vi "BB_Local Sense Test_v3.vi"(7 "error in (no error)":errorcluster, 10 "Control Board VISA":refnum<visa-resource-name>) -> (0 "error out":errorcluster, 2 "Voltage Readings":dbl[][](array[numeric]), 3 "Pass?":bool)   [LabVIEW 2022 SP3]
panel:
  in  "LocalSenseRelayTask":refnum<k21>="BTS_LocalSenseRelays"
  out "MSE Array":dbl[](array[numeric])
  out "Message OUT":string
  in  "Message IN":string
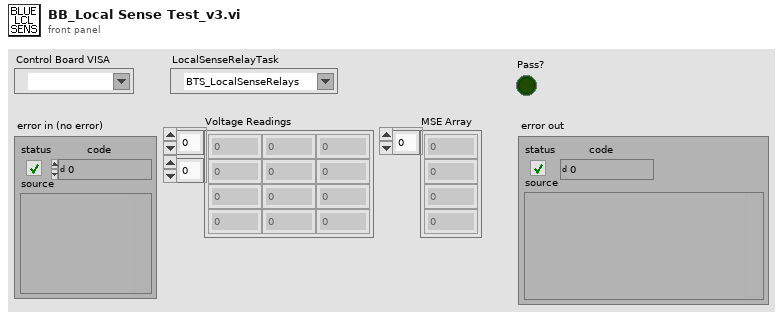
[diagram p1: front panel]
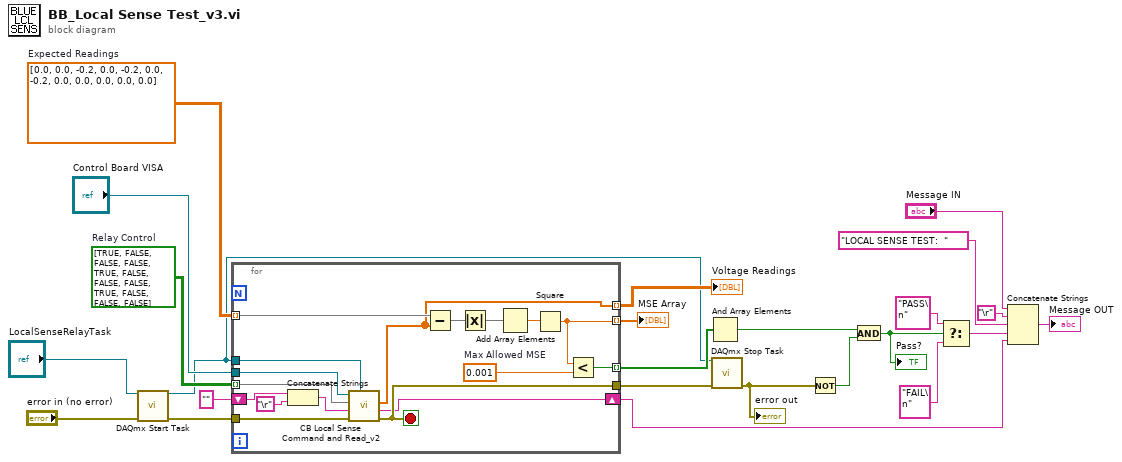
[diagram p0: block diagram]
diagram:
  w7 = dbl[][] [[0.0, 0.0, -0.2], [0.0, -0.2, 0.0], [-0.2, 0.0, 0.0], [0.0, 0.0, 0.0]]  # Expected Readings
  w23 = bool[][] [[TRUE, FALSE, FALSE], [FALSE, TRUE, FALSE], [FALSE, FALSE, TRUE], [FALSE, FALSE, FALSE]]  # Relay Control
  n1 = call <vilib>:"DAQmx Start Task.vi"("task/channels in"="LocalSenseRelayTask", "error in"="error in (no error)") -> ("task out"=w1:refnum<k21>, "error out"=w4:errorcluster)  [unwired: 12 in]
  n2 = for {
    tunnel: [w40] -> w3
    tunnel: w4 -> [w41]
    tunnel: w7 -> [w37] mode=indexing
    tunnel: [w34] -> w24 mode=indexing
    tunnel: w23 -> [w33] mode=indexing
    tunnel: [w32] -> w20 mode=indexing
    tunnel: [w31] -> w19 mode=indexing
    shift-right: [w30] -> w12
    shift-left: "" -> [w29]
    tunnel: "Control Board VISA" -> [w26]
    tunnel: w1 -> [w25]
    stop <- w40 stop-if-true
    w35 = 0.001  # Max Allowed MSE
    n3 = Concatenate Strings(w29, "\r") -> (w28:string)
    n4 = call "CB Local Sense Command and Read_v2.vi"("LocalSenseRelayTask"=w25, "error in (no error)"=w41, "Message IN"=w28, "Relay Control"=w33, "Control Board VISA"=w26) -> ("error out"=w40:errorcluster, "Message OUT"=w30:string, "Voltage Array"=w32:dbl[])  [unwired: 3 in, 1 out]
    n5 = Subtract(x=w37, y=w32) -> (x-y=w39:dbl[])
    n6 = Absolute Value(x=w39) -> (abs(x)=w38:dbl[])
    n7 = Add Array Elements(numeric array=w38) -> (sum=w36:dbl)
    n8 = Square(x=w36) -> (x^2=w31:dbl)
    n9 = Less?(x=w31, y=w35) -> (x < y?=w34:bool)
  }
  "Voltage Readings" <- w20
  "MSE Array" <- w19
  n10 = And Array Elements(Boolean array=w24) -> (logical AND=w22:bool)
  n11 = call <vilib>:"DAQmx Stop Task.vi"("task/channels in"=w1, "error in"=w3) -> ("error out"=w2:errorcluster)  [unwired: 12 in, 1 out]
  "error out" <- w2
  n12 = Not(x=w2) -> (.not. x?=w21:bool)
  n13 = And(x=w22, y=w21) -> (x .and. y?=w14:bool)
  "Pass?" <- w14
  n14 = Select(t="PASS\n", s=w14, f="FAIL\n") -> (s? t:f=w13:string)
  n15 = Concatenate Strings("Message IN", "\r", "LOCAL SENSE TEST:  ", w13, w12) -> (→"Message OUT":string)
